vi "Get Reserved Names.vi"() -> (2 "reserved names":string[](array[string])=["InstrumentStudioPluginSDK"])   [LabVIEW 2021, in "InstrumentStudio Plug-In Editor.lvlib"]
uses:
  InstrumentStudio Plug-In Editor.lvlib
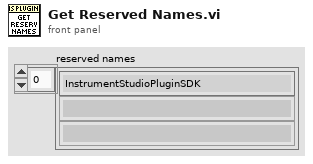
[diagram p1: front panel]
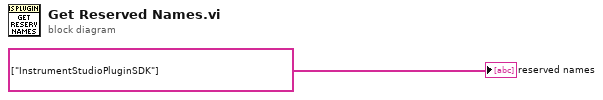
[diagram p0: block diagram]
diagram:
  "reserved names" <- string[] ["InstrumentStudioPluginSDK"] ("Libraries from MeasurementLink Runtime")
